vi "GFITS_CloseIfValid.vi"(5 "log":bool, 7 "logfile":path, 8 "error in (no error)":errorcluster, 11 "fref in":u64) -> (0 "error out":errorcluster, 3 "fref  out":u64)   [LabVIEW 2016]
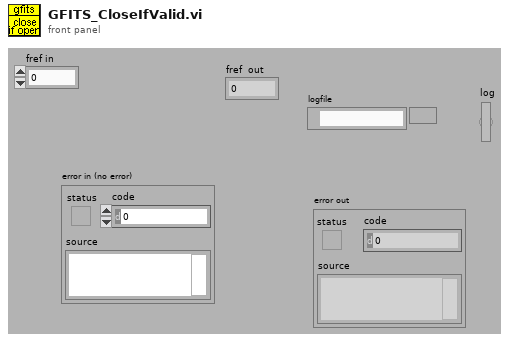
[diagram p1: front panel]
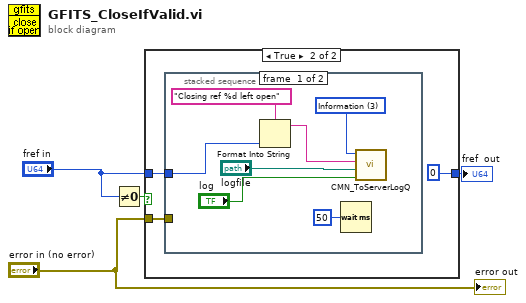
[diagram p0: block diagram]
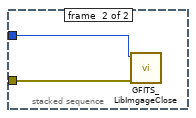
[diagram p3: hidden frame]
diagram:
  n1 = Not Equal To 0?(x="fref in") -> (x != 0?=w4:bool)
  n2 = case shown="True" w4 {
    tunnel: "fref in" -> [w5 w8]
    tunnel: "error in (no error)" -> [_ w7]
    tunnel: [w5 u64 0] -> w2
    frame False {
    }
    frame True {
      n3 = stacked-sequence {
        tunnel: w8 -> [w12 w17]
        tunnel: w7 -> [_ w16]
        frame #0 {
          w13 = u16 3 items=["command", "imediateReply", "Callback Reply", "Information", "none"] ("type")
          n4 = Format Into String(format string="Closing ref %d left open", w12) -> (resulting string=w10:string)  [unwired: 2 in, 1 out]
          n5 = Wait (ms)(milliseconds to wait=u32 50) -> ()  [unwired: 1 out]
          n6 = call "CMN_ToServerLogQ.vi"("Log"="log", "file"="logfile", "string"=w10, "type"=w13) -> ()  [unwired: 2 in, 5 out]
        }
        frame #1 {
          n7 = call "GFITS_LibImgageClose.vi"("error in (no error)"=w16, "fd"=w17) -> ()  [unwired: 1 in, 9 out]
        }
      }
    }
  }
  "fref  out" <- w2
  "error out" <- "error in (no error)"
